vi "Basic BC Test.vi"   [LabVIEW 2016]
uses:
  1553 Component/1553 Component.lvclass
  Bus Controller/Bus Controller.lvclass
  Bus Controller/TypeDefs/Bus Controller Configuration.ctl
  Frames & Messages/Major Frame/Major Frame.lvclass
  PPLs/FPGA Interface.lvlibp/FPGA Interface/FPGA Interface.lvclass
  D:/SVN/Products/SLSC/Multichannel 1553 Module/Software/Source Code/Driver (Windows)/1553 SubComponent/1553 SubComponent.lvclass
types:
  T1 = typedef "SLSC 1553 API.lvlib/Bus Controller.lvclass/Bus Controller Configuration.ctl" = cluster{"BC Timeout":u16, "BC Retry":bool, "BC Second Retry":bool, "BC Retry Alt Bus":bool, "BC Second Retry Alt Bus":bool, "BC Retry on Status Bit":bool, "Msg Error No Data Valid":bool, "Busy Status No Data Valid":bool, "Msg Gap Timer":bool, "Watchdog Timer":bool, "Time Tag Sync":bool, "Even Time Tag Sync":bool, "Gap Check":bool, "Broadcast Mask Enable":bool}
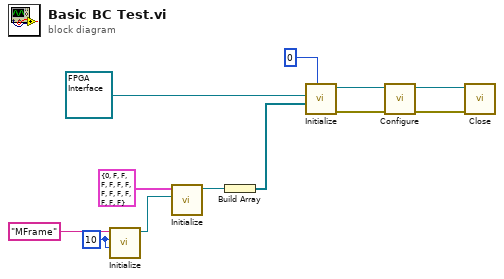
[diagram p0: block diagram]
diagram:
  w1 = u16 10 ("Major Frame Time (us)")
  n1 = call "Initialize.vi"("Minor Frame Time (us)"=w1, 10:w1, "ID"="MFrame") -> ("Major Frame out"=w5:refnum<class "Major Frame.lvclass">)  [unwired: 7 in, 1 out]
  n2 = call "Initialize.vi"("Major Frame"=w5, "Configuration"=T1 {"BC Timeout"=0, "BC Retry"=FALSE, "BC Second Retry"=FALSE, "BC Retry Alt Bus"=FALSE, "BC Second Retry Alt Bus"=FALSE, "BC Retry on Status Bit"=FALSE, "Msg Error No Data Valid"=FALSE, "Busy Status No Data Valid"=FALSE, "Msg Gap Timer"=FALSE, "Watchdog Timer"=FALSE, "Time Tag Sync"=FALSE, "Even Time Tag Sync"=FALSE, "Gap Check"=FALSE, "Broadcast Mask Enable"=FALSE}) -> ("Bus Controller out"=w3:refnum<class "Bus Controller.lvclass">)  [unwired: 8 in, 1 out]
  n3 = Build Array(w3) -> (w2:refnum<class "Bus Controller.lvclass">[])
  n4 = call "Initialize.vi"("Component ID (1-8)"=u8 0 ("Component ID"), "SubComponents"=w2, "FPGA Interface"=refnum<class "FPGA Interface.lvclass"> refnum) -> ("error out"=w9:errorcluster, "1553 Component out"=w11:refnum<class "1553 Component.lvclass">)  [unwired: 7 in]
  n5 = call-dynamic "Configure.vi"("error in (no error)"=w9, "1553 Component in"=w11) -> ("error out"=w8:errorcluster, "1553 Component out"=w10:refnum<class "1553 Component.lvclass">)  [unwired: 8 in]
  n6 = call-dynamic "Close.vi"("error in (no error)"=w8, "1553 Component in"=w10) -> ()  [unwired: 9 in, 1 out]
